vi "Diff Filter.vi"(10 "Diff Points":i32, 11 "Raw EC Data in":i16[][](array[numeric])) -> (3 "Raw EC Data out":i16[][](array[numeric]))   [LabVIEW 2017]
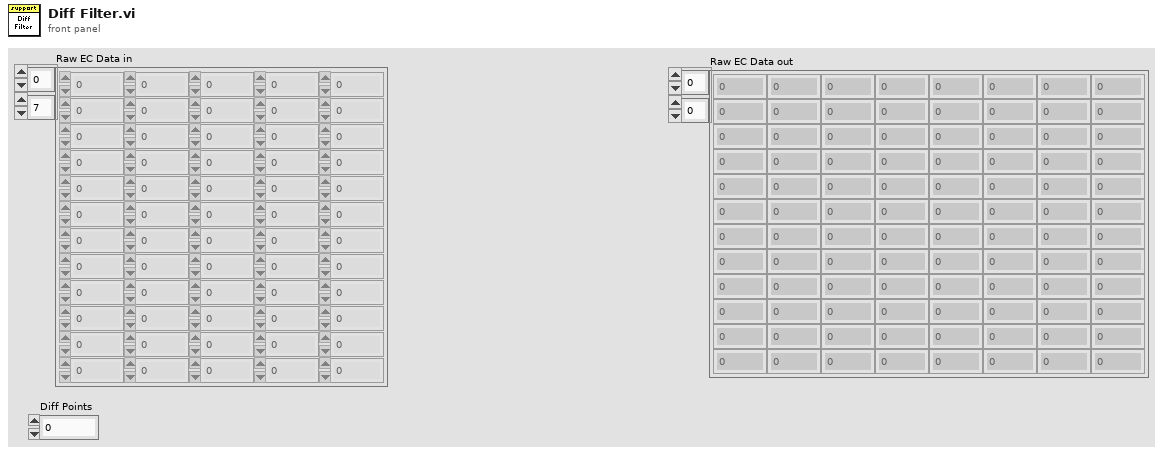
[diagram p1: front panel]
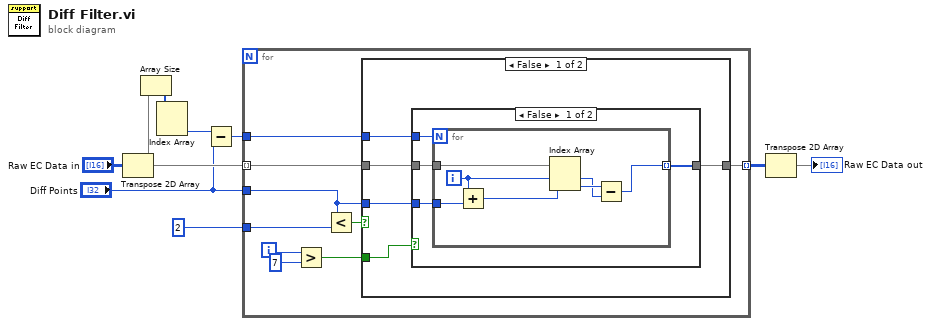
[diagram p0: block diagram]
diagram:
  n1 = Transpose 2D Array(2D array="Raw EC Data in") -> (transposed array=w7:i16[][])
  n2 = Array Size(array=w7) -> (size(s)=w8:i32[])
  n3 = Index Array(array=w8) -> (element #2=w2:i32)  [unwired: 2 in, 1 out]
  n4 = Subtract(x=w2, y="Diff Points") -> (x-y=w1:i32)
  n5 = for {
    tunnel: w7 -> [w18] mode=indexing
    tunnel: w1 -> [w16]
    tunnel: [w17] -> w6 mode=indexing
    tunnel: 2 ("y") -> [w14]
    tunnel: "Diff Points" -> [w13]
    i -> [w12]
    n6 = Greater?(x=w12, y=7) -> (0:w10:bool)
    n7 = Less?(x=w13, y=w14) -> (x < y?=w15:bool)
    n8 = case shown="False" w15 {
      tunnel: w18 -> [w23 w36]
      tunnel: [w22 w36] -> w17
      tunnel: w16 -> [w20 _]
      tunnel: w13 -> [w21 _]
      tunnel: w10 -> [w19 _]
      frame False {
        n9 = case shown="False" w19 {
          tunnel: w23 -> [w27 w35]
          tunnel: [w26 w35] -> w22
          tunnel: w21 -> [w25 _]
          tunnel: w20 -> [w24 _]
          frame False {
            n10 = for {
              N: w24 -> [_]
              tunnel: w27 -> [w34]
              tunnel: w25 -> [w32]
              tunnel: [w29] -> w26 mode=indexing
              i -> [w33]
              n11 = Add(x=w33, y=w32) -> (x+y=w28:i32)
              n12 = Index Array(array=w34, index #1=w33, index #2=w28) -> (element #1=w30:i16, element #2=w31:i16)
              n13 = Subtract(x=w31, y=w30) -> (x-y=w29:i16)
            }
          }
          frame True {
          }
        }
      }
      frame True {
      }
    }
  }
  n14 = Transpose 2D Array(2D array=w6) -> (transposed array=→"Raw EC Data out":i16[][])
